vi "Patch data preview-Obtain single cycle data.vi"(9 "Channel to load":enum16{"Red", "Green"}(ring), 10 "Global cycle number among all trials":i32, 11 "Register cluster":T1) -> (0 "error out":errorcluster, 3 "Data from single channel single cycle":dbl[](array[numeric]))   [LabVIEW 2017]
uses:
  Typedefs/Patch viewer internal cluster.ctl
  <vilib>/vision/Image Controls.llb/IMAQ Image.ctl
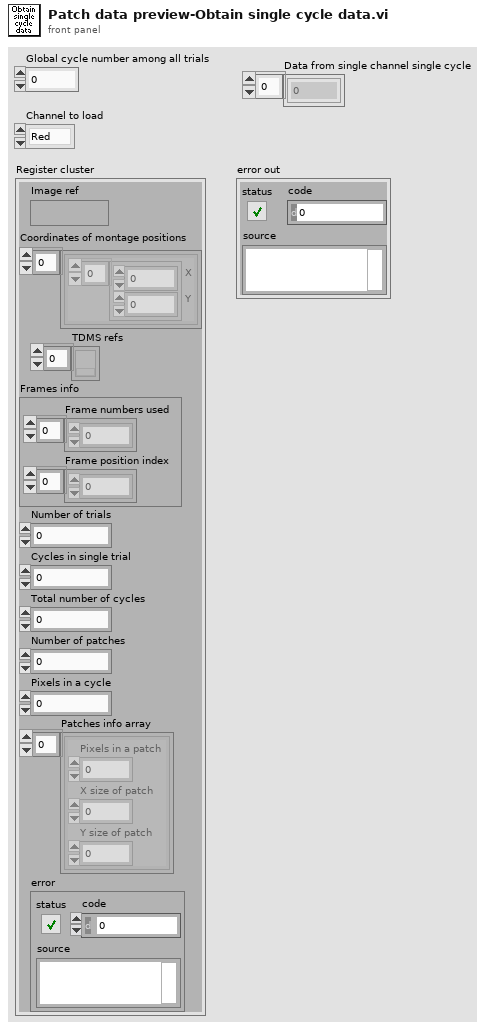
[diagram p1: front panel]
types:
  T1 = typedef "Patch viewer internal cluster.ctl" = cluster{"Image ref":T2, "Coordinates of montage positions":cluster{"X\n\nY":i32[]}[], "TDMS refs":refnum<k34>[], "Frames info":cluster{"Frame numbers used":i32[], "Frame position index":i32[]}, "Number of trials":i32, "Cycles in single trial":i32, "Total number of cycles":i32, "Number of patches":i32, "Pixels in a cycle":i32, "Patches info array":cluster{"Pixels in a patch":i32, "X size of patch":i32, "Y size of patch":i32}[], "error":errorcluster}
  T2 = typedef "IMAQ Image.ctl" = refnum<image>
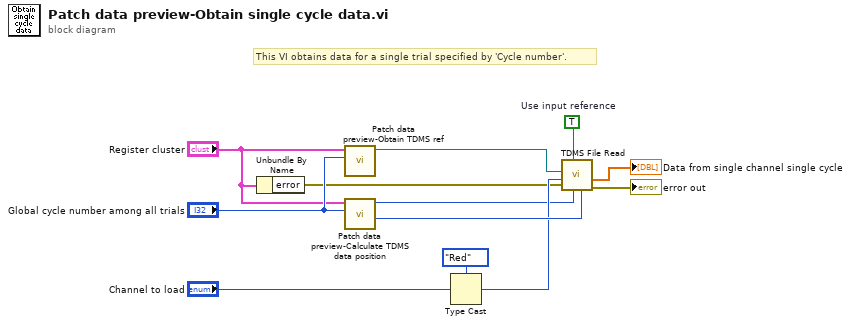
[diagram p0: block diagram]
diagram:
  w1 = TRUE  # Use input reference
  # "This VI obtains data for a single trial specified by 'Cycle number'."
  n1 = Unbundle By Name("Register cluster") -> ("error"=w6:errorcluster)
  n2 = call "Patch data preview-Obtain TDMS ref.vi"("Cycle number"="Global cycle number among all trials", "Register cluster"="Register cluster") -> ("TDMS ref"=w4:refnum<k34>)  [unwired: 8 in, 1 out]
  n3 = call "Patch data preview-Calculate TDMS data position.vi"("Global cycle number among all trials"="Global cycle number among all trials", "Register cluster"="Register cluster") -> ("Cycle's data length"=w12:i64, "Cycle's data start index in current trial"=w2:i64)  [unwired: 8 in]
  n4 = Type Cast(type=enum16{"Red", "Green", "Both"}."Red" ("Channel to load"), x="Channel to load") -> (*(type *) &x=w8:enum16{"Red", "Green", "Both"})
  n5 = call "TDMS File Read.vi"("count (-1: all)"=w12, "offset (0)"=w2, "Use input reference (F)"=w1, "Error In"=w6, "Channel to load"=w8, "tdms file ref"=w4) -> ("Error Out"=→"error out":errorcluster, "Single channel data"=→"Data from single channel single cycle":dbl[])  [unwired: 2 in, 2 out]
